vi "DFD NStage MRate Filtering.vi"   [LabVIEW 2017, in "NI_DigFilterLicensed.lvlib"]
doc: "Filters a signal continuously with a multistage multirate filter. Wire data to the <B>signal in</B> input to determine the polymorphic instance to use or manually select the instance."
uses:
  <vilib>/addons/Digital Filter Design/NI_DigFilterLicensed.lvlib
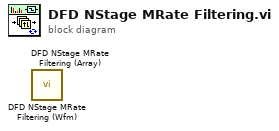
[diagram p0: block diagram]
diagram:
  n1 = call <vilib>:"DFD NStage MRate Filtering (Wfm).vi"() -> ()  [unwired: 10 in, 2 out]
  n2 = call <vilib>:"DFD NStage MRate Filtering (Array).vi"() -> ()  [unwired: 10 in, 2 out]
